vi "MsgExists.vi"(9 "Msg Type":string, 11 "Msg Path":path) -> (0 "Package/Msg":string, 2 "Msg Exists?":bool)   [LabVIEW 2014]
doc: "check to see if a message exists in a given message package\nreturns message with the package name"
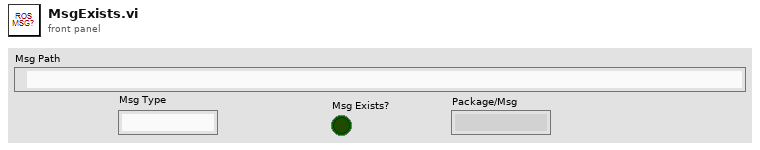
[diagram p1: front panel]
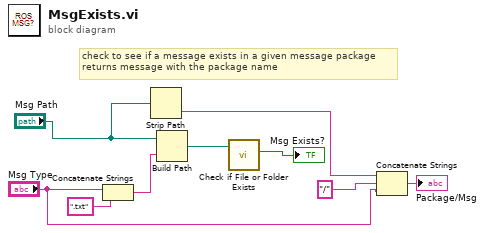
[diagram p0: block diagram]
diagram:
  # "check to see if a message exists in a given message package\nreturns message with the package name"
  n1 = Concatenate Strings("Msg Type", ".txt" ("string")) -> (w7:string)
  n2 = Strip Path(path="Msg Path") -> (name=w4:string)  [unwired: 1 out]
  n3 = Build Path(base path="Msg Path", name or relative path=w7) -> (appended path=w8:path)
  n4 = call <vilib>:"Check if File or Folder Exists.vi"("path"=w8) -> ("file or folder exists?"=→"Msg Exists?":bool)  [unwired: 8 in, 2 out]
  n5 = Concatenate Strings(w4, "/" ("string"), "Msg Type") -> (→"Package/Msg":string)
